vi "Lake_shore_set.vi"() -> ()   [LabVIEW 2015]
panel:
  in  "Heater On/Off":bool
  in  "Temp Ramping Rate (K/min) 2":dbl=10.0
  in  "Heater Range":enum16{"Off", "Low", "Medium", "High"}(ring)
  in  "Set temperature (K)":dbl=4.5
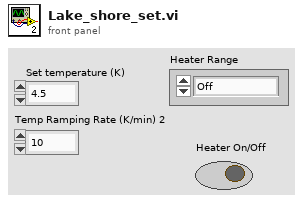
[diagram p1: front panel]
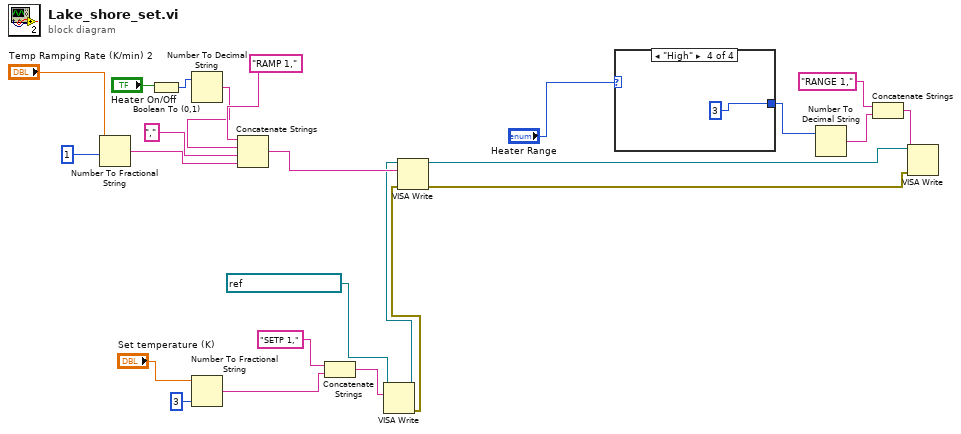
[diagram p0: block diagram]
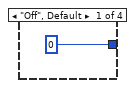
[diagram p2: hidden frame]
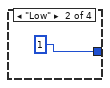
[diagram p3: hidden frame]
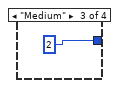
[diagram p4: hidden frame]
diagram:
  n1 = Number To Fractional String(number="Temp Ramping Rate (K/min) 2", precision (6)=i16 1) -> (F-format string=w6:string)  [unwired: 2 in]
  n2 = Boolean To (0,1)(Boolean="Heater On/Off") -> (0, 1=w9:i16)
  n3 = Number To Decimal String(number=w9) -> (decimal integer string=w7:string)  [unwired: 1 in]
  n4 = Number To Fractional String(number="Set temperature (K)", precision (6)=i16 3) -> (F-format string=w22:string)  [unwired: 2 in]
  n5 = Concatenate Strings("RAMP 1," ("string"), w7, "," ("string"), w6) -> (w11:string)
  n6 = Concatenate Strings("SETP 1," ("write buffer"), w22) -> (w20:string)
  n7 = VISA Write(VISA resource name=refnum<visa-resource-name> "GPIB0::11::INSTR", write buffer=w20) -> (VISA resource name out=w3:refnum<visa-resource-name>, error out=w4:errorcluster)  [unwired: 1 in, 1 out]
  n8 = VISA Write(VISA resource name=w3, write buffer=w11, error in (no error)=w4) -> (VISA resource name out=w2:refnum<visa-resource-name>, error out=w1:errorcluster)  [unwired: 1 out]
  n9 = case shown="\"High\"" "Heater Range" {
    tunnel: [0 1 2 3] -> w17
    frame "Off", Default {
    }
    frame "Low" {
    }
    frame "Medium" {
    }
    frame "High" {
    }
  }
  n10 = Number To Decimal String(number=w17) -> (decimal integer string=w16:string)  [unwired: 1 in]
  n11 = Concatenate Strings("RANGE 1," ("write buffer"), w16) -> (w15:string)
  n12 = VISA Write(VISA resource name=w2, write buffer=w15, error in (no error)=w1) -> ()  [unwired: 3 out]
